vi "picture.vi"() -> ()   [LabVIEW 2022 SP3]
panel:
  in  "Save File Path":path
  out "Image":T1(plugin-control)
  in  "Open File Path":path
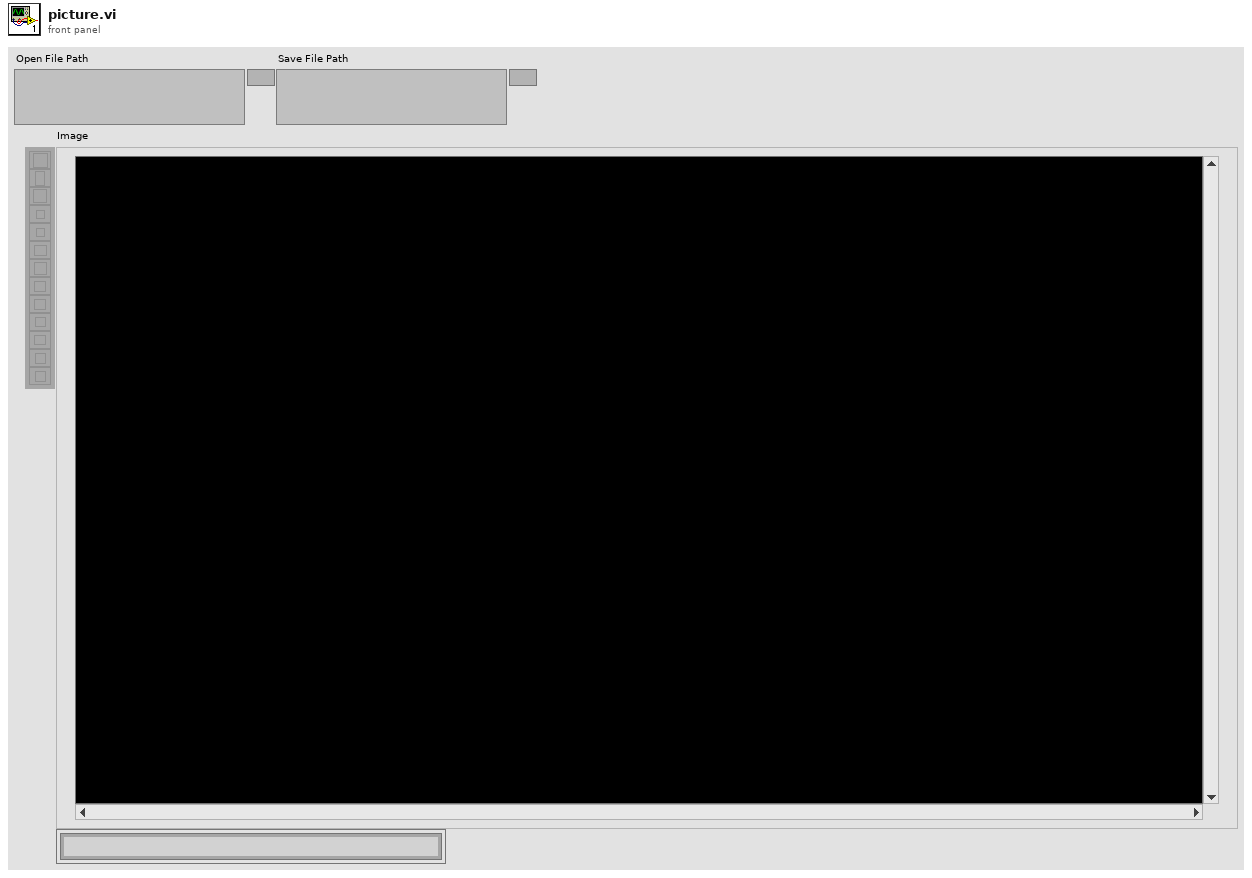
[diagram p1: front panel]
types:
  T1 = typedef "IMAQ Image.ctl" = refnum<image>
  T2 = typedef "Image Type" = u32
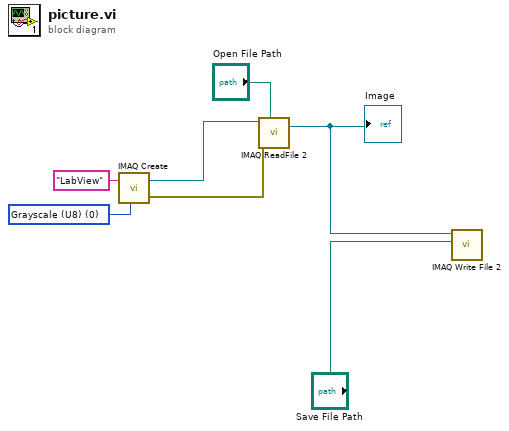
[diagram p0: block diagram]
diagram:
  w3 = T2 0 items=["Grayscale (U8)", "Grayscale (I16)", "Grayscale (SGL)", "Complex (CSG)", "RGB (U32)", "HSL (U32)", "RGB (U64)", "Grayscale (U16)"] ("Image Type")
  n1 = call "IMAQ Create"("Image Name"="LabView", "Image Type"=w3) -> ("New Image"=w7:T1, "error out"=w6:errorcluster)  [unwired: 3 in]
  n2 = call "IMAQ ReadFile 2"("File Path"="Open File Path", "error in (no error)"=w6, "Image"=w7) -> ("Image Out"=w1:T1)  [unwired: 4 in, 4 out]
  "Image" <- w1
  n3 = call-poly "IMAQ Write File 2"("File Path"="Save File Path", "Image"=w1) -> ()  [unwired: 8 in, 2 out]
